vi "Get Menu Item VI.vi"(7 "Menu Item":string, 8 "error in (no error)":errorcluster, 9 "GUID":string, 10 "Item Ref":T1 format="%.0x", 11 "System Explorer Dispatcher Implementation in":refnum<class "System Explorer Dispatcher.lvclass">) -> (0 "error out":errorcluster, 2 "menu item reference":refnum<vi>, 3 "System Explorer Dispatcher Implementation out":refnum<class "System Explorer Dispatcher.lvclass">)   [LabVIEW 2020, in "Ballard ARINC 429 System Explorer.lvlib" / "Implementation.lvlib" / "System Explorer Dispatcher.lvclass"]
uses:
  System Explorer Dispatcher.lvclass
  <vilib>/NI VeriStand/Custom Device API/Custom Device Item Ref.ctl
  Scripting/Constants.vi
  Scripting/Ballard ARINC 429 Scripting.lvlib
  Implementation.lvlib
  <vilib>/NI VeriStand/Custom Device API/Custom Device API.lvlib
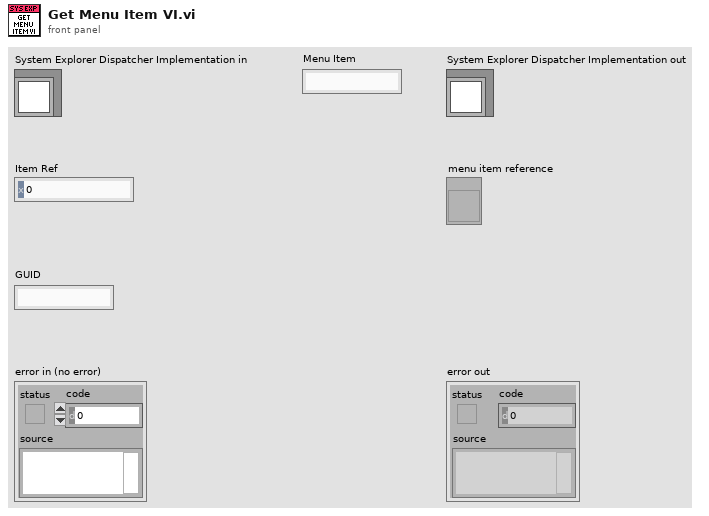
[diagram p1: front panel]
types:
  T1 = typedef "Custom Device API.lvlib/Custom Device Item Ref.ctl" = u64
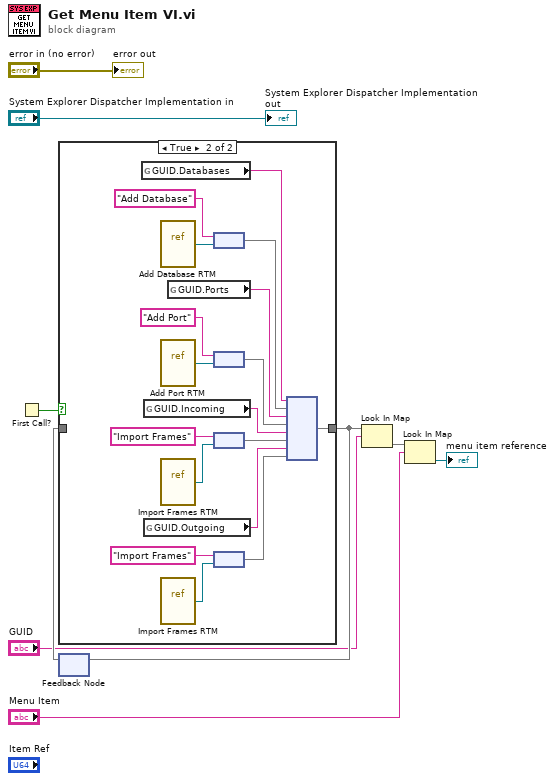
[diagram p0: block diagram]
diagram:
  n1 = First Call?() -> (First Call?: T/F=w1:bool)
  n2 = feedback #1() -> (w7:map{string, map{string, refnum<vi>}})  [unwired: 1 in]
  n3 = case shown="True" w1 {
    tunnel: [w10 w27] -> w8
    tunnel: w7 -> [w10 _]
    frame False {
    }
    frame True {
      n4 = global read "Constants.vi" "GUID.Databases"() -> (w26:string)
      n5 = global read "Constants.vi" "GUID.Incoming"() -> (w16:string)
      n6 = global read "Constants.vi" "GUID.Outgoing"() -> (w12:string)
      n7 = vi-ref "Add Database RTM.vi"() -> (w22:refnum<vi>)
      n8 = vi-ref "Add Port RTM.vi"() -> (w19:refnum<vi>)
      n9 = vi-ref "Import Frames RTM.vi"() -> (w18:refnum<vi>)
      n10 = vi-ref "Import Frames RTM.vi"() -> (w13:refnum<vi>)
      n11 = global read "Constants.vi" "GUID.Ports"() -> (w25:string)
      n12 = node("Add Database", w22) -> (w24:map{string, refnum<vi>})
      n13 = node("Add Port", w19) -> (w20:map{string, refnum<vi>})
      n14 = node("Import Frames", w18) -> (w15:map{string, refnum<vi>})
      n15 = node("Import Frames", w13) -> (w11:map{string, refnum<vi>})
      n16 = node(w26, w24, w25, w20, w16, w15, w12, w11) -> (w27:map{string, map{string, refnum<vi>}})
    }
  }
  n17 = feedback-in #1(w8) -> ()
  n18 = Look In Map(map=w8, key="GUID") -> (value=w5:map{string, refnum<vi>})  [unwired: 1 in, 1 out]
  n19 = Look In Map(map=w5, key="Menu Item") -> (value=→"menu item reference":refnum<vi>)  [unwired: 1 in, 1 out]
  "error out" <- "error in (no error)"
  "System Explorer Dispatcher Implementation out" <- "System Explorer Dispatcher Implementation in"
